vi "Plug_in_data_global.vi"() -> ()   [LabVIEW 2011]
panel:
  in  "FFID Bkgnd Values":dbl[](array[numeric])
  in  "Templated Results header":string
  in  "Block Header":string
  in  "Server Channels to log":string[](array[string])
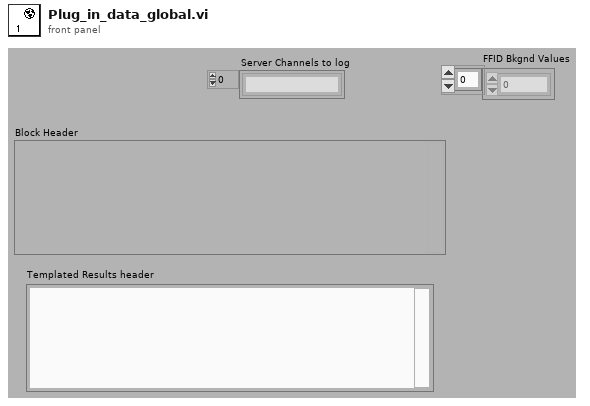
[diagram p1: front panel]
diagram:
